vi "I2C Grove 64x128OLED_SSD1315_Graph.vi"() -> ()   [LabVIEW 2020]
uses:
  CTI/I2C Number.ctl
  CTI/GPIO Number.ctl
  CTI/Session/Session.lvclass
  CTI-Peripheral/Grove I2C LCD/Grove I2C LCD.lvclass
  CTI/VisaComms/VisaComms.lvclass
  CTI/CTI.lvlib
panel:
  out "error out":errorcluster
  in  "Port":refnum<visa-resource-name>="COM4"
  in  "String":string="Hello LabVIEW!"
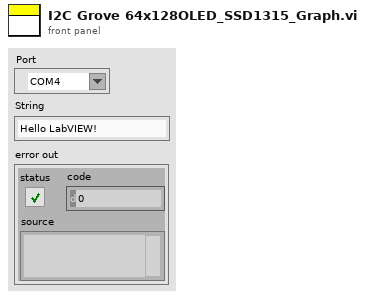
[diagram p1: front panel]
types:
  T1 = typedef "CTI.lvlib/GPIO Number.ctl" = i8
  T2 = typedef "CTI.lvlib/I2C Number.ctl" = i8
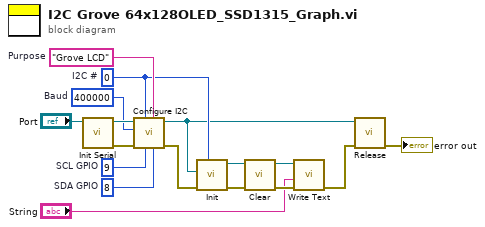
[diagram p0: block diagram]
diagram:
  w9 = T1 8  # SDA GPIO
  w10 = T1 9  # SCL GPIO
  w11 = "Grove LCD"  # Purpose
  w2 = T2 0  # I2C #
  w12 = u32 400000  # Baud
  n1 = call "Init Serial.vi"("VISA resource name in"="Port") -> ("error out"=w13:errorcluster, "Session"=w14:refnum<class "Session.lvclass">)  [unwired: 8 in, 1 out]
  n2 = call "Configure I2C.vi"("SDA GPIO"=w9, "Purpose (\"I2C\")"=w11, "SCL GPIO"=w10, "I2C #"=w2, "error in (no error)"=w13, "Baud"=w12, "Session in"=w14) -> ("error out"=w8:errorcluster, "Session out"=w1:refnum<class "Session.lvclass">)  [unwired: 3 in]
  n3 = call "Init.vi"("I2C #"=w2, "error in (no error)"=w8, "Session In"=w1) -> ("error out"=w7:errorcluster, "Grove I2C LCD out"=w6:refnum<class "Grove I2C LCD.lvclass">)  [unwired: 7 in]
  n4 = call-dynamic "Clear.vi"("error in (no error)"=w7, "Character LCD in"=w6) -> ("error out"=w17:errorcluster, "Character LCD out"=w5:refnum<class "Grove I2C LCD.lvclass">)  [unwired: 8 in]
  n5 = call-dynamic "Write Text.vi"("error in (no error)"=w17, "Text"="String", "Character LCD in"=w5) -> ("error out"=w3:errorcluster)  [unwired: 7 in, 1 out]
  n6 = call-dynamic "Release.vi"("error in (no error)"=w3, "Session in"=w1) -> ("error out"=→"error out":errorcluster)  [unwired: 9 in]
